vi "PhotonPoseEstimator_SetRobotToCamera.vi"(9 "RobotToCameraTransform3d":T10={"TRANSLATION3D"={"X"=0.0, "Y"=0.0, "Z"=0.0}, "ROTATION3D"={"Q_quaternion"={"R"=1.0, "V"=[0.0, 0.0, 0.0]}}, "XF"=FALSE} {"TRANSLATION3D"."Z" format="%14.3f"; "TRANSLATION3D"."Y" format="%14.3f"; "TRANSLATION3D"."X" format="%14.3f"}, 11 "PhotonPoseEstimator":T1={"LastPose"={"Translation3d"={"X"=0.0, "Y"=0.0, "Z"=0.0}, "Rotation3d"={"Q_quaternion"={"R"=1.0, "V"=[0.0, 0.0, 0.0]}}}, "ReferencePose"={"Translation3d"={"X"=0.0, "Y"=0.0, "Z"=0.0}, "Rotation3d"={"Q_quaternion"={"R"=1.0, "V"=[0.0, 0.0, 0.0]}}}, "FieldTags"={"AprilTagMap"={}, "FieldLength"=0.0, "FieldWidth"=0.0, "OriginPosition "=enum."kBlueAllianceWallRightSide,", "OriginPose3d"={"Translation3d"={"X"=0.0, "Y"=0.0, "Z"=0.0}, "Rotation3d"={"Q_quaternion"={"R"=1.0, "V"=[0.0, 0.0, 0.0]}}}}, "PhotonPoseStrategy"=enum."LOWEST_AMBIGUITY", "Camera"="", "RobotToCamera"={"TRANSLATION3D"={"X"=0.0, "Y"=0.0, "Z"=0.0}, "ROTATION3D"={"Q_quaternion"={"R"=1.0, "V"=[0.0, 0.0, 0.0]}}, "XF"=FALSE}, "ReportedErrors"=[], "HighestAmbiguity"=10.0} {"RobotToCamera"."TRANSLATION3D"."Z" format="%14.3f"; "RobotToCamera"."TRANSLATION3D"."Y" format="%14.3f"; "RobotToCamera"."TRANSLATION3D"."X" format="%14.3f"; "FieldTags"."OriginPose3d"."Translation3d"."Z" format="%14.3f"; "FieldTags"."OriginPose3d"."Translation3d"."Y" format="%14.3f"; "FieldTags"."OriginPose3d"."Translation3d"."X" format="%14.3f"; "ReferencePose"."Translation3d"."Z" format="%14.3f"; "ReferencePose"."Translation3d"."Y" format="%14.3f"; "ReferencePose"."Translation3d"."X" format="%14.3f"; "LastPose"."Translation3d"."Z" format="%14.3f"; "LastPose"."Translation3d"."Y" format="%14.3f"; "LastPose"."Translation3d"."X" format="%14.3f"}) -> (3 "out PhotonPoseEstimator":T1={"LastPose"={"Translation3d"={"X"=0.0, "Y"=0.0, "Z"=0.0}, "Rotation3d"={"Q_quaternion"={"R"=1.0, "V"=[0.0, 0.0, 0.0]}}}, "ReferencePose"={"Translation3d"={"X"=0.0, "Y"=0.0, "Z"=0.0}, "Rotation3d"={"Q_quaternion"={"R"=1.0, "V"=[0.0, 0.0, 0.0]}}}, "FieldTags"={"AprilTagMap"={}, "FieldLength"=0.0, "FieldWidth"=0.0, "OriginPosition "=enum."kBlueAllianceWallRightSide,", "OriginPose3d"={"Translation3d"={"X"=0.0, "Y"=0.0, "Z"=0.0}, "Rotation3d"={"Q_quaternion"={"R"=1.0, "V"=[0.0, 0.0, 0.0]}}}}, "PhotonPoseStrategy"=enum."LOWEST_AMBIGUITY", "Camera"="", "RobotToCamera"={"TRANSLATION3D"={"X"=0.0, "Y"=0.0, "Z"=0.0}, "ROTATION3D"={"Q_quaternion"={"R"=1.0, "V"=[0.0, 0.0, 0.0]}}, "XF"=FALSE}, "ReportedErrors"=[], "HighestAmbiguity"=10.0} {"RobotToCamera"."TRANSLATION3D"."Z" format="%14.3f"; "RobotToCamera"."TRANSLATION3D"."Y" format="%14.3f"; "RobotToCamera"."TRANSLATION3D"."X" format="%14.3f"; "FieldTags"."OriginPose3d"."Translation3d"."Z" format="%14.3f"; "FieldTags"."OriginPose3d"."Translation3d"."Y" format="%14.3f"; "FieldTags"."OriginPose3d"."Translation3d"."X" format="%14.3f"; "ReferencePose"."Translation3d"."Z" format="%14.3f"; "ReferencePose"."Translation3d"."Y" format="%14.3f"; "ReferencePose"."Translation3d"."X" format="%14.3f"; "LastPose"."Translation3d"."Z" format="%14.3f"; "LastPose"."Translation3d"."Y" format="%14.3f"; "LastPose"."Translation3d"."X" format="%14.3f"})   [LabVIEW 2019, in "PhotonVisionLib.lvlib"]
doc: "Set the current strategy being used by the PhotonPoseEstimator.\n\nInputs: \n -- PhotonVisionPoseEstimator -- cluster -- The estimator.\n -- PhotonPoseStrategy -- enum -- Current strategy being used by the Photon Pose Estimator. Current strategies include:\n LOWEST_AMBIGUITY -- Choose the Pose with the lowest ambiguity\n CLOSEST_TO_CAMERA_HEIGHT -- Choose the Pose which is closest to the camera height.\n CLOSEST_TO_REFERENCE_POSE -- Choose the Pose which is closest to a set Reference position.\n CLOSEST_TO_LAST_POSE -- Choose the Pose which is closest to the last pose calculated\n AVERAGE_BEST_TARGETS -- Weight average of acceptable targets based on ambiguity..\n\nOutputs:\n -- PhotonVisionPoseEstimator -- cluster -- The updated estimator."
uses:
  TypeDef/PhotonPoseEstimatorType.ctl
  <vilib>/Rock Robotics/WPI/ThirdParty/JAS_Junk/TrajLib/TypeDef/POSE3D.ctl
  <vilib>/Rock Robotics/WPI/ThirdParty/JAS_Junk/TrajLib/TypeDef/TRANSLATION3D.ctl
  <vilib>/Rock Robotics/WPI/ThirdParty/JAS_Junk/TrajLib/TypeDef/ROTATION3D.ctl
  <vilib>/Rock Robotics/WPI/ThirdParty/JAS_Junk/TrajLib/TypeDef/QUATERNION.ctl
  <vilib>/Rock Robotics/WPI/ThirdParty/JAS_Junk/TrajLib/TypeDef/AprilTagFieldLayout.ctl
  <vilib>/Rock Robotics/WPI/ThirdParty/JAS_Junk/TrajLib/TypeDef/AprilTag.ctl
  <vilib>/Rock Robotics/WPI/ThirdParty/JAS_Junk/TrajLib/Enum/AprilTagFieldLayoutOrignPosition_ENUM.ctl
  Enum/PhotonPoseStrategy_ENUM.ctl
  <vilib>/Rock Robotics/WPI/ThirdParty/JAS_Junk/TrajLib/TypeDef/TRANSFORM3D.ctl
  PhotonVisionLib.lvlib
  <vilib>/Rock Robotics/WPI/ThirdParty/JAS_Junk/TrajLib/Trajectory_Library.lvlib
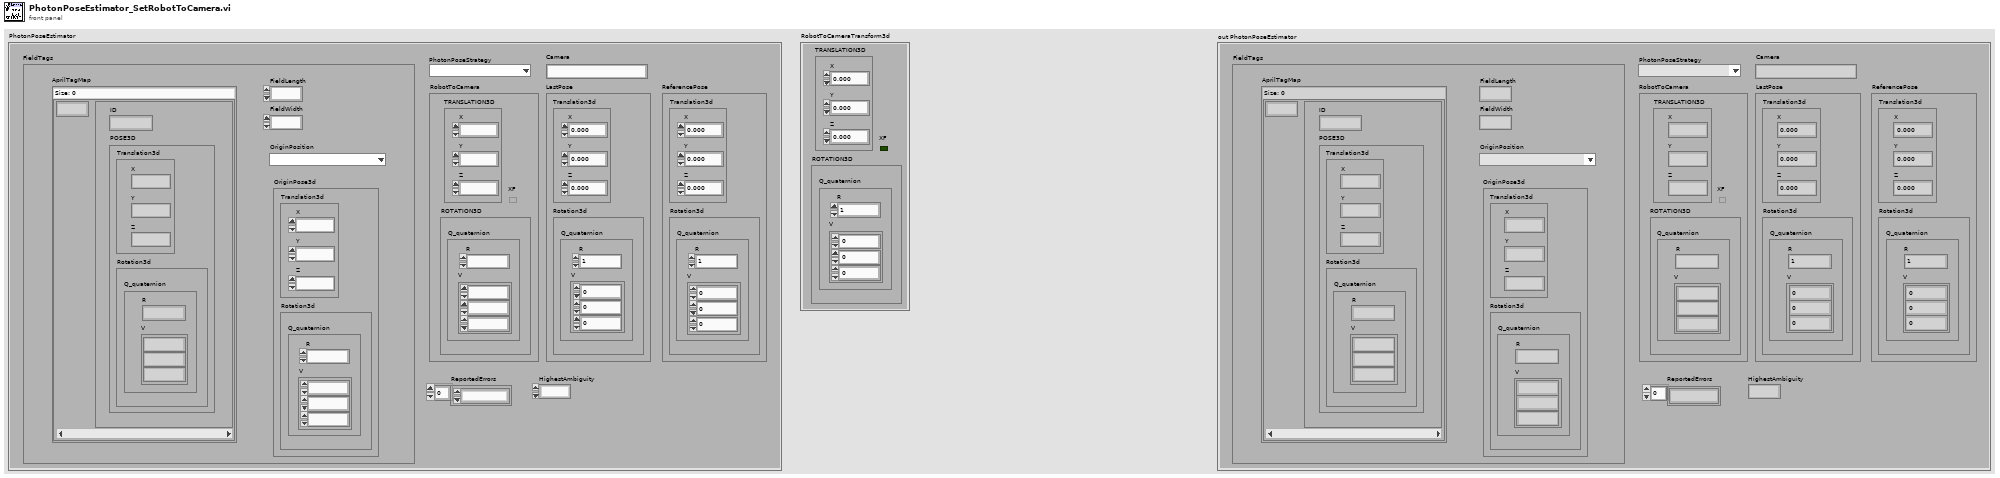
[diagram p1: front panel]
types:
  T1 = typedef "PhotonVisionLib.lvlib/PhotonPoseEstimatorType.ctl" = cluster{"LastPose":T2, "ReferencePose":T2, "FieldTags":T6, "PhotonPoseStrategy":T9, "Camera":string, "RobotToCamera":T10, "ReportedErrors":dbl[], "HighestAmbiguity":dbl}
  T2 = typedef "Trajectory_Library.lvlib/POSE3D.ctl" = cluster{"Translation3d":T3, "Rotation3d":T4}
  T3 = typedef "Trajectory_Library.lvlib/TRANSLATION3D.ctl" = cluster{"X":dbl, "Y":dbl, "Z":dbl}
  T4 = typedef "Trajectory_Library.lvlib/ROTATION3D.ctl" = cluster{"Q_quaternion":T5}
  T5 = typedef "Trajectory_Library.lvlib/QUATERNION.ctl" = cluster{"R":dbl, "V":dbl[]}
  T6 = typedef "Trajectory_Library.lvlib/AprilTagFieldLayout.ctl" = cluster{"AprilTagMap":map{i32, T7}, "FieldLength":dbl, "FieldWidth":dbl, "OriginPosition ":T8, "OriginPose3d":T2}
  T7 = typedef "Trajectory_Library.lvlib/AprilTag.ctl" = cluster{"ID":i32, "POSE3D":T2}
  T8 = typedef "Trajectory_Library.lvlib/AprilTagFieldLayoutOrignPosition_ENUM.ctl" = enum16{"kBlueAllianceWallRightSide,", "kRedAllianceWallRightSide,"}
  T9 = typedef "PhotonVisionLib.lvlib/PhotonPoseStrategy_ENUM.ctl" = enum16{"LOWEST_AMBIGUITY", "CLOSEST_TO_CAMERA_HEIGHT", "CLOSEST_TO_REFERENCE_POSE", "CLOSEST_TO_LAST_POSE", "AVERAGE_BEST_TARGETS"}
  T10 = typedef "Trajectory_Library.lvlib/TRANSFORM3D.ctl" = cluster{"TRANSLATION3D":T3, "ROTATION3D":T4, "XF":bool}
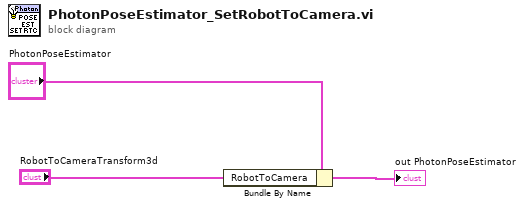
[diagram p0: block diagram]
diagram:
  n1 = Bundle By Name(cluster="PhotonPoseEstimator", "RobotToCamera"="RobotToCameraTransform3d") -> (→"out PhotonPoseEstimator":T1)
